vi "Example.vi"() -> ()   [LabVIEW 2019]
uses:
  firebase.lvclass
  Filtering Parameters--cluster.ctl
  1fc7c40c-8b97-48a6-9ebc-2eea49d1469b.vi
  c716dd23-e44b-4cc0-bcf0-07ea465b1354.vi
  <vilib>/JDP Science/JSONtext/JSON text to Variant.vi
  <vilib>/JDP Science/JSONtext/LVClass Serializer/JSONtext LVClass Serializer.lvclass
  <vilib>/JDP Science/JSONtext/JSONtext.lvlib
panel:
  in  "Tab Control":enum32{"Log IN/Sign IN", "POST", "GET"}(tab)
  in  "Password":string
  in  "Email":string
  in  "Log In":bool
  in  "Sign In":bool
  in  "Volts":dbl(knob) scale=0.0..1000.0
  in  "Enable":bool
  in  "Post":bool
  out "data":T1 {"date" format="%<%x %.3X>T"}
  in  "Get Newest":bool
  out "Last 5":T2(array[cluster]) {"date" format="%<%x %.3X>T"}
  in  "Get Last 5":bool
  in  "Exit":bool
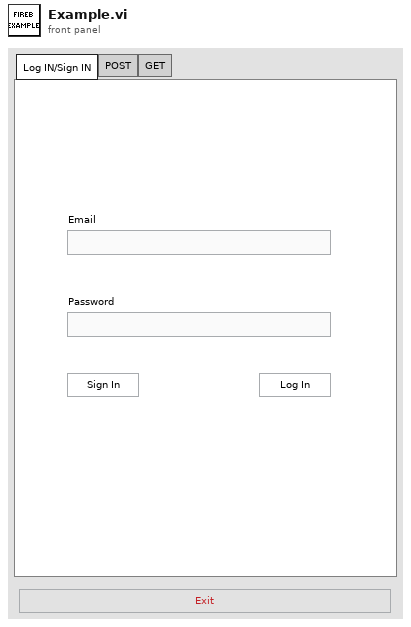
[diagram p1: front panel]
types:
  T1 = cluster{"Volts":dbl, "Enable":bool, "date":timestamp}
  T2 = cluster{"Volts":dbl, "Enable":bool, "date":timestamp}[]
  T3 = typedef "firebase.lvclass/Filtering Parameters--cluster.ctl" = cluster{"Filtering Param":string, "Argument":string}
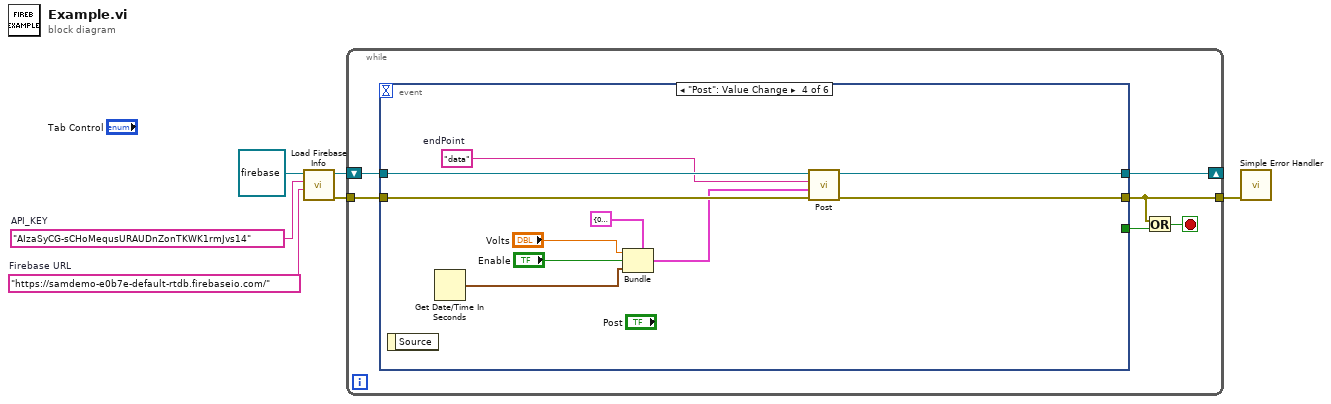
[diagram p0: block diagram]
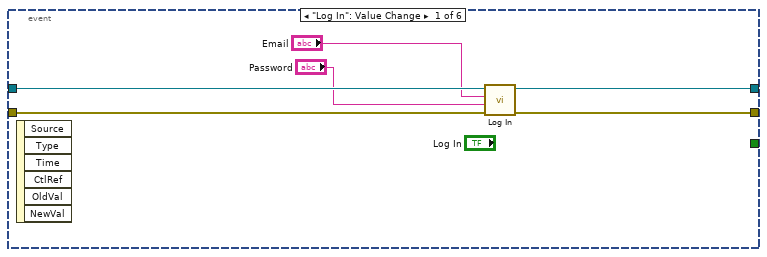
[diagram p2: hidden frame]
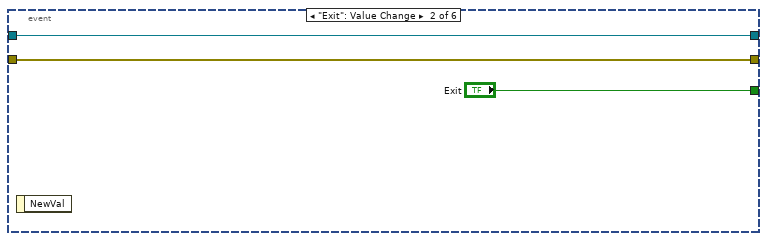
[diagram p3: hidden frame]
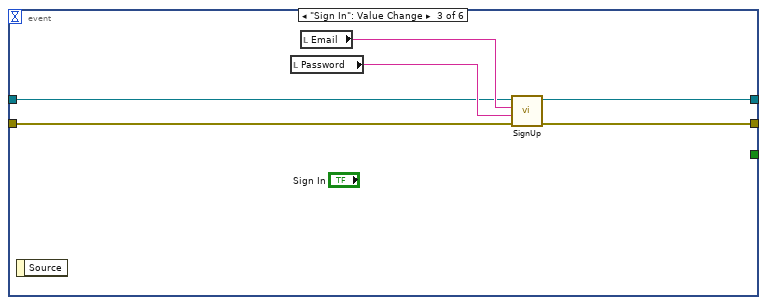
[diagram p4: hidden frame]
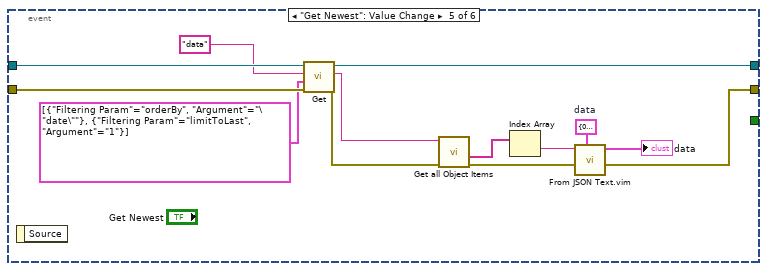
[diagram p5: hidden frame]
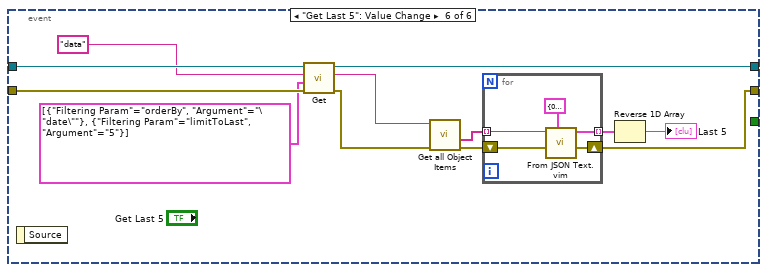
[diagram p6: hidden frame]
diagram:
  w2 = "AIzaSyCG-sCHoMequsURAUDnZonTKWK1rmJvs14"  # API_KEY
  w3 = "https://samdemo-e0b7e-default-rtdb.firebaseio.com/"  # Firebase URL
  n1 = call "Load Firebase Info.vi"("Firebase URL"=w3, "API_KEY"=w2, "firebase in"=refnum<class "firebase.lvclass"> refnum ("firebase.lvclass")) -> ("error out"=w6:errorcluster, "firebase out"=w1:refnum<class "firebase.lvclass">)  [unwired: 7 in]
  n2 = while {
    tunnel: w6 -> [w12]
    tunnel: [w11] -> w5
    shift-right: [w9] -> _
    shift-left: w1 -> [w10]
    stop <- w7 stop-if-true
    n3 = event shown="[3] \"Post\": Value Change" {
      selector: _ -> [_ _ _ _ _ _]
      dyn-events: _ -> [_ _ _ _ _ _]
      timeout: _ -> [_ _ _ _ _ _]
      tunnel: w12 -> [w18 w21 w27 w37 w50 w62]
      tunnel: w10 -> [w16 w19 w23 w35 w46 w58]
      tunnel: [w17 w21 w26 w36 w47 w59] -> w11
      tunnel: [w13 w19 w22 w34 w45 w57] -> w9
      tunnel: [_ "Exit" _ _ _ _] -> w8
      event "Log In": Value Change {
        n4 = event-data() -> ()  [unwired: 1 in, 6 out]
        n5 = call-dynamic "Log In.vi"("error in"=w18, "password"="Password", "email"="Email", "firebase in"=w16) -> ("error out"=w17:errorcluster, "firebase out"=w13:refnum<class "firebase.lvclass">)  [unwired: 6 in]
      }
      event "Exit": Value Change {
        n6 = event-data() -> ()  [unwired: 1 in, 1 out]
      }
      event "Sign In": Value Change {
        n7 = event-data() -> ()  [unwired: 1 in, 1 out]
        n8 = local read "Password"() -> (w25:string)
        n9 = local read "Email"() -> (w24:string)
        n10 = call-dynamic "SignUp.vi"("error in"=w27, "password"=w25, "email"=w24, "firebase in"=w23) -> ("error out"=w26:errorcluster, "firebase out"=w22:refnum<class "firebase.lvclass">)  [unwired: 6 in]
      }
      event "Post": Value Change {
        w33 = "data"  # endPoint
        n11 = event-data() -> ()  [unwired: 1 in, 1 out]
        n12 = Get Date/Time In Seconds() -> (seconds since 1Jan1904=w32:timestamp)
        n13 = Bundle(cluster=T1 {"Volts"=0.0, "Enable"=FALSE, "date"=timestamp(0 s since 1904-01-01)}, "Volts"="Volts", "Enable"="Enable", "date"=w32) -> (w31:T1)
        n14 = call-dynamic "Post.vi"("error in"=w37, "Anything"=w31, "endPoint"=w33, "firebase in"=w35) -> ("error out"=w36:errorcluster, "firebase out"=w34:refnum<class "firebase.lvclass">)  [unwired: 5 in, 1 out]
      }
      event "Get Newest": Value Change {
        w42 = T1 {"Volts"=0.0, "Enable"=FALSE, "date"=timestamp(0 s since 1904-01-01)}  # data
        n15 = event-data() -> ()  [unwired: 1 in, 1 out]
        n16 = call-dynamic "Get.vi"("error in"=w50, "Filtering Params"=T3[] [{"Filtering Param"="orderBy", "Argument"="\"date\""}, {"Filtering Param"="limitToLast", "Argument"="1"}], "endPoint"="data", "firebase in"=w46) -> ("error out"=w49:errorcluster, "Json String"=w39:string, "firebase out"=w45:refnum<class "firebase.lvclass">)  [unwired: 5 in]
        n17 = call <vilib>:"Get all Object Items.vi"("error in (no error)"=w49, "JSON"=w39) -> ("error out"=w48:errorcluster, "<JSON>"=w41:string[])  [unwired: 6 in, 2 out]
        n18 = Index Array(array=w41) -> (element=w40:string)  [unwired: 1 in]
        n19 = call "From JSON Text.vim"("Data Type and Default Value"=w42, "error in (no error)"=w48, "JSON"=w40) -> ("error out"=w47:errorcluster, "Data out"=→"data":T1)  [unwired: 7 in]
      }
      event "Get Last 5": Value Change {
        n20 = event-data() -> ()  [unwired: 1 in, 1 out]
        n21 = call-dynamic "Get.vi"("error in"=w62, "Filtering Params"=T3[] [{"Filtering Param"="orderBy", "Argument"="\"date\""}, {"Filtering Param"="limitToLast", "Argument"="5"}], "endPoint"="data", "firebase in"=w58) -> ("error out"=w60:errorcluster, "Json String"=w53:string, "firebase out"=w57:refnum<class "firebase.lvclass">)  [unwired: 5 in]
        n22 = call <vilib>:"Get all Object Items.vi"("error in (no error)"=w60, "JSON"=w53) -> ("error out"=w61:errorcluster, "<JSON>"=w54:string[])  [unwired: 6 in, 2 out]
        n23 = for {
          tunnel: w54 -> [w64] mode=indexing
          shift-right: [w66] -> w59
          shift-left: w61 -> [w67]
          tunnel: [w63] -> w52 mode=indexing
          n24 = call "From JSON Text.vim"("Data Type and Default Value"=T1 {"Volts"=0.0, "Enable"=FALSE, "date"=timestamp(0 s since 1904-01-01)} ("data"), "error in (no error)"=w67, "JSON"=w64) -> ("error out"=w66:errorcluster, "Data out"=w63:T1)  [unwired: 7 in]
        }
        n25 = Reverse 1D Array(array=w52) -> (reversed array=→"Last 5":T2)
      }
    }
    n26 = Or(x=w11, y=w8) -> (x .or. y?=w7:bool)
  }
  n27 = call <vilib>:"Simple Error Handler.vi"("error in (no error)"=w5) -> ()  [unwired: 4 in, 5 out]
